vi "GlobalFileInfo.vi"() -> ()   [LabVIEW 2010]
panel:
  in  "Data Type":u32
  in  "Y Dim":u32
  in  "X Dim":u32
  in  "File Handle":u32
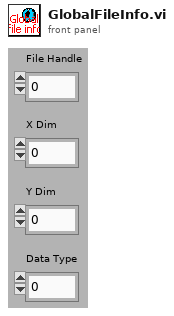
[diagram p1: front panel]
diagram:
